vi "Get Name From Enum.vi"(8 "error in (no error)":errorcluster, 10 "Channel Enum":u16=65535, 11 "CIFChannelMng in":refnum<class "CIFChannelMng.lvclass">) -> (0 "error out":errorcluster, 2 "Channel Name out":string, 3 "CIFChannelMng out":refnum<class "CIFChannelMng.lvclass">)   [LabVIEW 2021, in "CIFChannelMng.lvclass"]
uses:
  CIFChannelMng.lvclass
  CIFChannelMng.lvclass/CIFChannelMng.ctl
  CIFClocks/Typedef/Errors.ctl
  CIFCore/Common/Utilities/Append Error Location.vi
  CIFCore/Common/CIFCoreCommon.lvlib
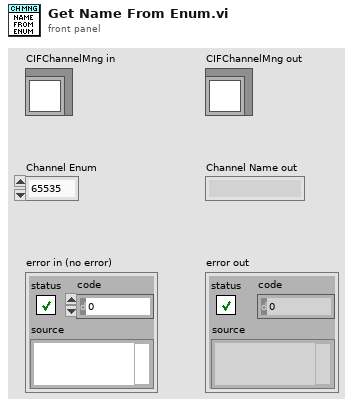
[diagram p1: front panel]
types:
  T1 = typedef "CIFCoreCommon.lvlib/Errors.ctl" = enum16{"Invalid Clock ID", "Long Sleep", "gRPC Server Not Found", "Config Parse", "Timestamp Wrap", "Delayed Execution", "Duplicate Channel", "Missing Channel", "Incorrect Type", "Unregistered Enum"}
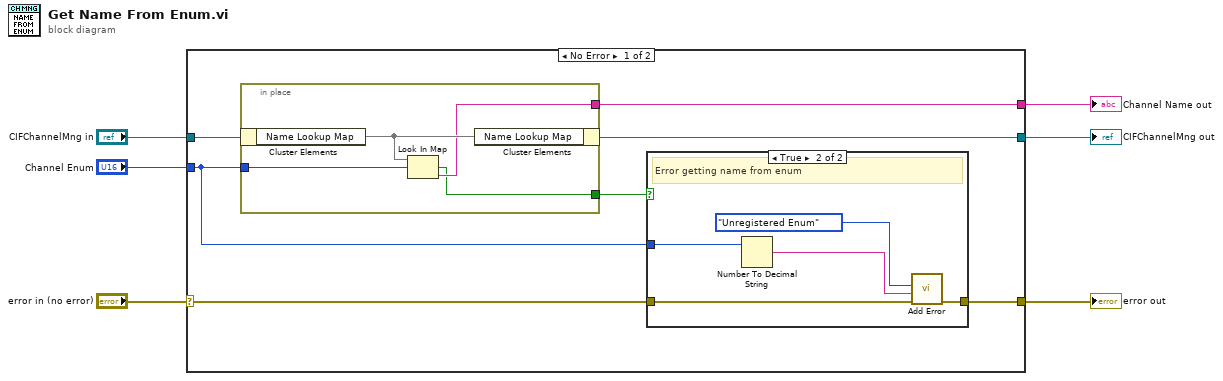
[diagram p0: block diagram]
diagram:
  n1 = case shown="No Error" "error in (no error)" {
    selector: "error in (no error)" -> [w11 w25]
    tunnel: [w10 w25] -> w5
    tunnel: [w9 w24] -> w3
    tunnel: "CIFChannelMng in" -> [w8 w24]
    tunnel: "Channel Enum" -> [w13 _]
    tunnel: [w12 _] -> w1
    frame No Error {
      n2 = in-place {
        in-place-border: w13 -> [w16]
        in-place-border: [w15] -> w12
        in-place-border: [w14] -> w7
        n3 = in-place-cluster #1(w8) -> ("Name Lookup Map"=w17:map{u16, string})
        n4 = Look In Map(map=w17, key=w16) -> (key not found?=w14:bool, value=w15:string)  [unwired: 1 in]
        n5 = in-place-cluster #1("Name Lookup Map"=w17) -> (w9:refnum<class "CIFChannelMng.lvclass">)
      }
      n6 = case shown="True" w7 {
        tunnel: w11 -> [w18 w23]
        tunnel: [w18 w22] -> w10
        tunnel: w13 -> [_ w20]
        frame False {
          # "no error"
        }
        frame True {
          # "Error getting name from enum"
          n7 = Number To Decimal String(number=w20) -> (decimal integer string=w21:string)  [unwired: 1 in]
          n8 = call "Add Error.vi"("error in (no error)"=w23, "String to Append"=w21, "Error"=Errors."Unregistered Enum") -> ("error out"=w22:errorcluster)  [unwired: 8 in]
        }
      }
    }
    frame Error {
    }
  }
  "error out" <- w5
  "CIFChannelMng out" <- w3
  "Channel Name out" <- w1
